vi "testFailureReturnsProvidedError.vi"() -> ()   [LabVIEW 2017, in "TestFailure.Tests.lvlib"]
uses:
  TestFailure.Tests.lvlib
  Test/Test.lvclass
  12e4e40a-799c-4c2f-8a04-e85da1adceba.vi
  <vilib>/Utility/error.llb/Error Cluster From Error Code.vi
  <vilib>/ErrorRing/Error Ring.xnode
  Constraint/IsEqual/IsEqual.lvclass
  TestFailure/TestFailure.lvclass
panel:
  out "error out":errorcluster
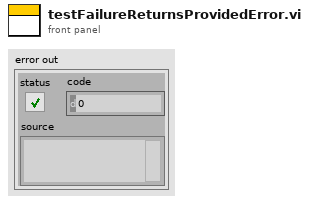
[diagram p1: front panel]
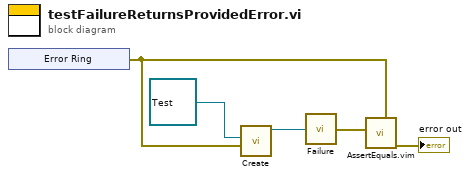
[diagram p0: block diagram]
diagram:
  n1 = xnode "Error Ring"() -> ("error out"=w2:errorcluster)
  n2 = call "Create.vi"("Failure"=w2, "Test"=refnum<class "Test.lvclass"> refnum ("TestCase")) -> ("TestFailure"=w5:refnum<class "TestFailure.lvclass">)  [unwired: 8 in, 1 out]
  n3 = call "Failure.vi"("TestFailure In"=w5) -> ("Failure"=w3:errorcluster)
  n4 = call "AssertEquals.vim"("Expected"=w2, "Actual"=w3) -> ("error out"=→"error out":errorcluster)  [unwired: 9 in]
